vi "Run Test.vi"(8 "error in (no error)":errorcluster, 11 "Test Template in":refnum<class "Load Defaults.lvclass">) -> (0 "error out":errorcluster, 1 "Positions":i32[](array[numeric]), 2 "Tests Passed":bool[](array[boolean]), 3 "Test Template out":refnum<class "Load Defaults.lvclass">, 5 "Fail Codes":string[](array[string]))   [LabVIEW 2015, in "Load Defaults.lvclass"]
uses:
  Load Defaults.lvclass
  Test Class/Test Class.lvclass
  Classes/Application/Class/Application.lvclass
  Classes/Parameter Loader/Class/Parameter Loader.lvclass
  <vilib>/Cree, Inc/Cree Test Framework/Classes/Base Objects/Base Class/Base Class/Base Class.lvclass
  Driver Test/Driver Test.lvclass
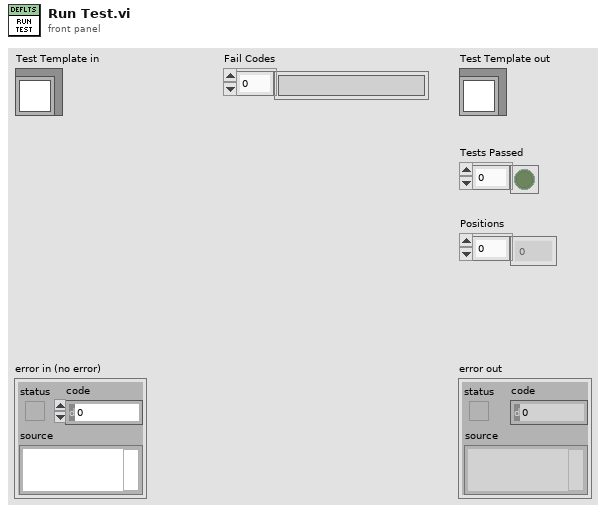
[diagram p1: front panel]
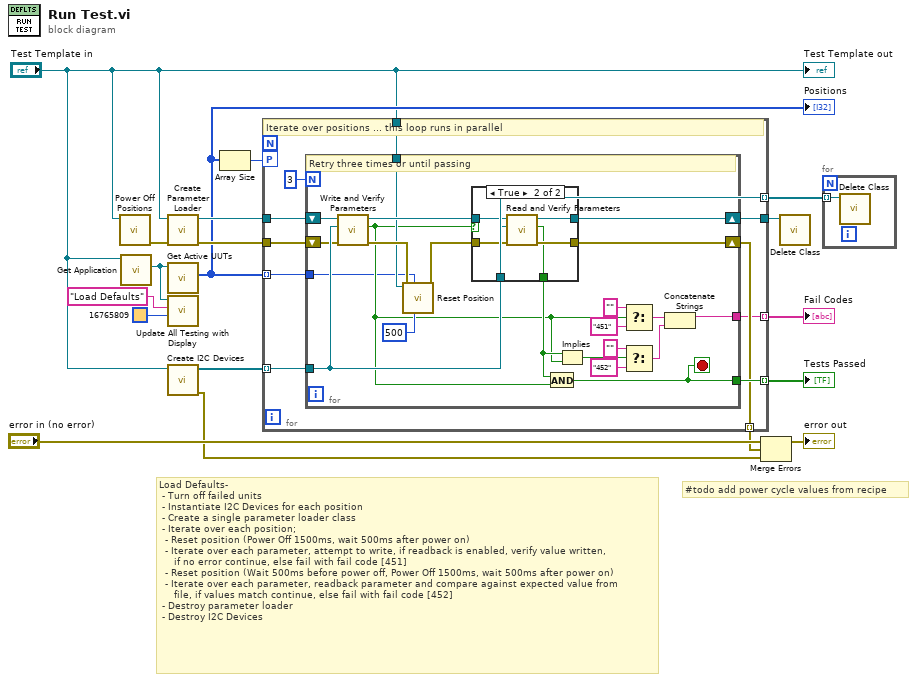
[diagram p0: block diagram]
diagram:
  # "#todo add power cycle values from recipe"
  # "Load Defaults-\n\t- Turn off failed units\n\t- Instantiate I2C Devices for each position\n\t- Create a single parameter loader class\n\t- Iterate over each position;\n\t\t- Reset position (Power Off 1500ms, wait 500ms after power on)\n\t\t- Iterate over each parameter, attempt to write, if readback is enabled, verify value written, \n     if no error continue, else fail with fail code [451]\n\t\t- Reset position (Wait 500ms before power off, Power Off 1500ms, wait 500ms after power on)\n\t\t- Iterate over each parameter, readback parameter and compare against expected value from \n     file, if values match continue, else fail with fail code [452]\n\t- Destroy parameter loader\n\t- Destroy I2C Devices"
  n1 = call "Power Off Positions.vi"("Driver Test"="Test Template in") -> ("error out"=w8:errorcluster)  [unwired: 10 in]
  n2 = call "Get Application.vi"("Test Class in"="Test Template in") -> ("Application.lvlib:Application.lvclass"=w3:refnum<class "Application.lvclass">)  [unwired: 9 in, 1 out]
  n3 = call "Create Parameter Loader.vi"("Error in"=w8, "Test Template in"="Test Template in") -> ("Error out"=w13:errorcluster, "Parameter Loader out"=w14:refnum<class "Parameter Loader.lvclass">)  [unwired: 8 in]
  n4 = call "Get Active UUTs.vi"("Application in"=w3) -> ("Active Positions"=w4:u32[])  [unwired: 8 in, 2 out]
  "Positions" <- w4
  n5 = call "Update All Testing with Display.vi"("BG Color"=u32 16765809, "Message ('')"="Load Defaults", "Application in"=w3) -> ()  [unwired: 7 in, 2 out]
  n6 = call "Create I2C Devices.vi"("Driver Test in"="Test Template in") -> ("error out"=w7:errorcluster, "I2C Devices"=w6:refnum<class "NI-8451.lvclass">[])  [unwired: 9 in]
  n7 = Array Size(array=w4) -> (size(s)=w9:i32)
  n8 = for {
    workers-P: w9 -> [_]
    tunnel: w6 -> [w23] mode=indexing
    tunnel: [w27] -> w5 mode=indexing
    tunnel: w14 -> [w28]
    tunnel: [w26] -> w15 mode=indexing
    tunnel: w13 -> [w25]
    tunnel: w4 -> [w21] mode=indexing
    tunnel: [w24] -> w12
    tunnel: [w23] -> w11 mode=indexing
    tunnel: [w20] -> w10 mode=indexing
    tunnel: "Test Template in" -> [w22]
    # "Iterate over positions ... this loop runs in parallel"
    n9 = for {
      N: 3 -> [_]
      tunnel: [w36] -> w27
      tunnel: w23 -> [w43]
      tunnel: w22 -> [w38]
      tunnel: w21 -> [w31]
      tunnel: [w30] -> w20
      shift-right: [w44] -> w24
      shift-left: w28 -> [w47]
      shift-right: [w32] -> w26
      shift-left: w25 -> [w29]
      stop <- w36 stop-if-true
      # "Retry three times or until passing"
      n10 = call "Write and Verify Parameters.vi"("error in (no error)"=w29, "I2C Device.lvclass"=w43, "Parameter Loader in"=w47) -> ("error out"=w50:errorcluster, "Success"=w33:bool, "Parameter Loader out"=w48:refnum<class "Parameter Loader.lvclass">)  [unwired: 6 in]
      n11 = call "Reset Position.vi"("Wait Before Reset (0ms)"=u32 500 ("Wait Before Reset (0)"), "Position"=w31, "error in (no error)"=w50, "Driver Test"=w38) -> ("error out"=w49:errorcluster)  [unwired: 7 in]
      n12 = case shown="True" w33 {
        tunnel: w49 -> [w51 w58]
        tunnel: w48 -> [w52 w57]
        tunnel: [w51 w56] -> w32
        tunnel: [w52 w55] -> w44
        tunnel: w43 -> [_ w54]
        tunnel: [_ w53] -> w34
        frame False {
        }
        frame True {
          n13 = call "Read and Verify Parameters.vi"("error in (no error)"=w58, "I2C Device.lvclass"=w54, "Parameter Loader in"=w57) -> ("error out"=w56:errorcluster, "Success"=w53:bool, "Parameter Loader out"=w55:refnum<class "Parameter Loader.lvclass">)  [unwired: 6 in]
        }
      }
      n14 = And(x=w34, y=w33) -> (x .and. y?=w36:bool)
      n15 = Implies(1:w33, 2:w34) -> (0:w35:bool)
      n16 = Select(t="", s=w33, f="451") -> (s? t:f=w42:string)
      n17 = Select(t="", s=w35, f="452") -> (s? t:f=w39:string)
      n18 = Concatenate Strings(w42, w39) -> (w30:string)
    }
  }
  "Tests Passed" <- w5
  "Fail Codes" <- w10
  n19 = Merge Errors("error in (no error)", w15, w7) -> (→"error out":errorcluster)
  n20 = call <vilib>:"Delete Class.vi"("Base Class in"=w12) -> ()  [unwired: 9 in, 2 out]
  n21 = for {
    tunnel: w11 -> [w59] mode=indexing
    n22 = call <vilib>:"Delete Class.vi"("Base Class in"=w59) -> ()  [unwired: 9 in, 2 out]
  }
  "Test Template out" <- "Test Template in"
